vi "Build Array.vi"() -> ()   [LabVIEW 2024]
panel:
  out "Output array":dbl[](array[numeric])
  in  "Element to Insert":dbl
  in  "Index":i32
  in  "Insert":bool
  in  "?":bool
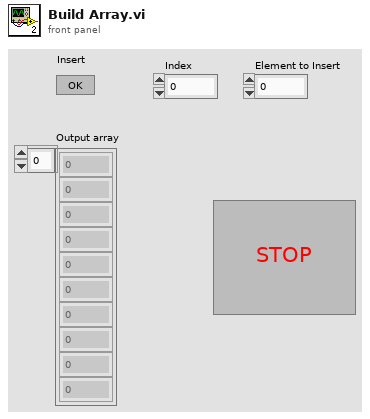
[diagram p1: front panel]
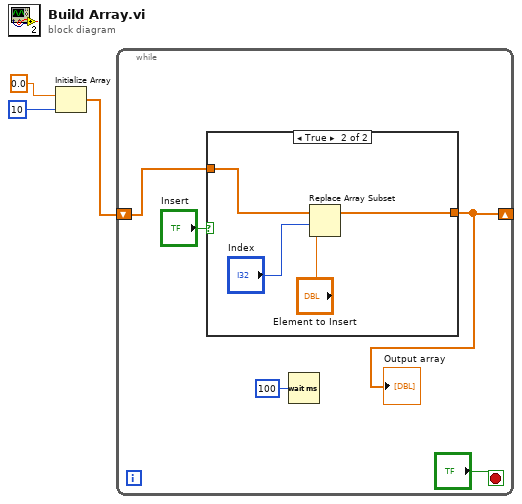
[diagram p0: block diagram]
diagram:
  n1 = Initialize Array(0.0 ("element"), 10 ("dimension size")) -> (w1:dbl[])
  n2 = while {
    shift-right: [w4] -> _
    shift-left: w1 -> [w5]
    stop <- "?" stop-if-true
    n3 = case shown="True" "Insert" {
      tunnel: w5 -> [w9 w11]
      tunnel: [w9 w10] -> w4
      frame False {
      }
      frame True {
        n4 = Replace Array Subset(array=w11, new element="Element to Insert", index="Index") -> (w10:dbl[])
      }
    }
    "Output array" <- w4
    n5 = Wait (ms)(milliseconds to wait=u32 100) -> ()  [unwired: 1 out]
  }
